vi "Write XML.vi"(9 "三级告警":string[][](array[string]), 10 "二级告警":string[][](array[string]), 11 "一级告警":string[][](array[string])) -> (0 "error out":errorcluster caption="错误输出", 3 "值":T1)   [LabVIEW 2016, in "Alarm interface.lvlib"]
uses:
  Alarm interface.lvlib
  <vilib>/Utility/xml.llb/Write to XML File(string).vi
panel:
  out "XML String":string caption="XML字符串"
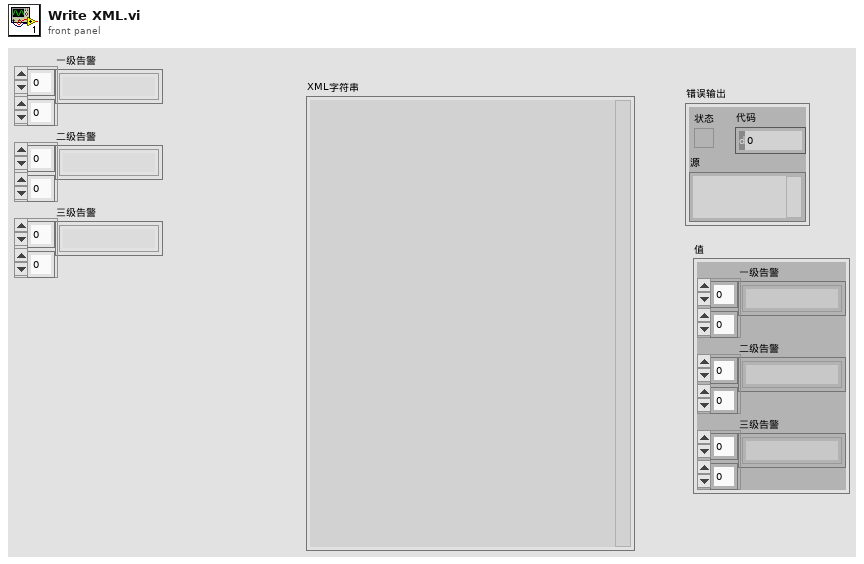
[diagram p1: front panel]
types:
  T1 = cluster{"一级告警":string[][], "二级告警":string[][], "三级告警":string[][]}
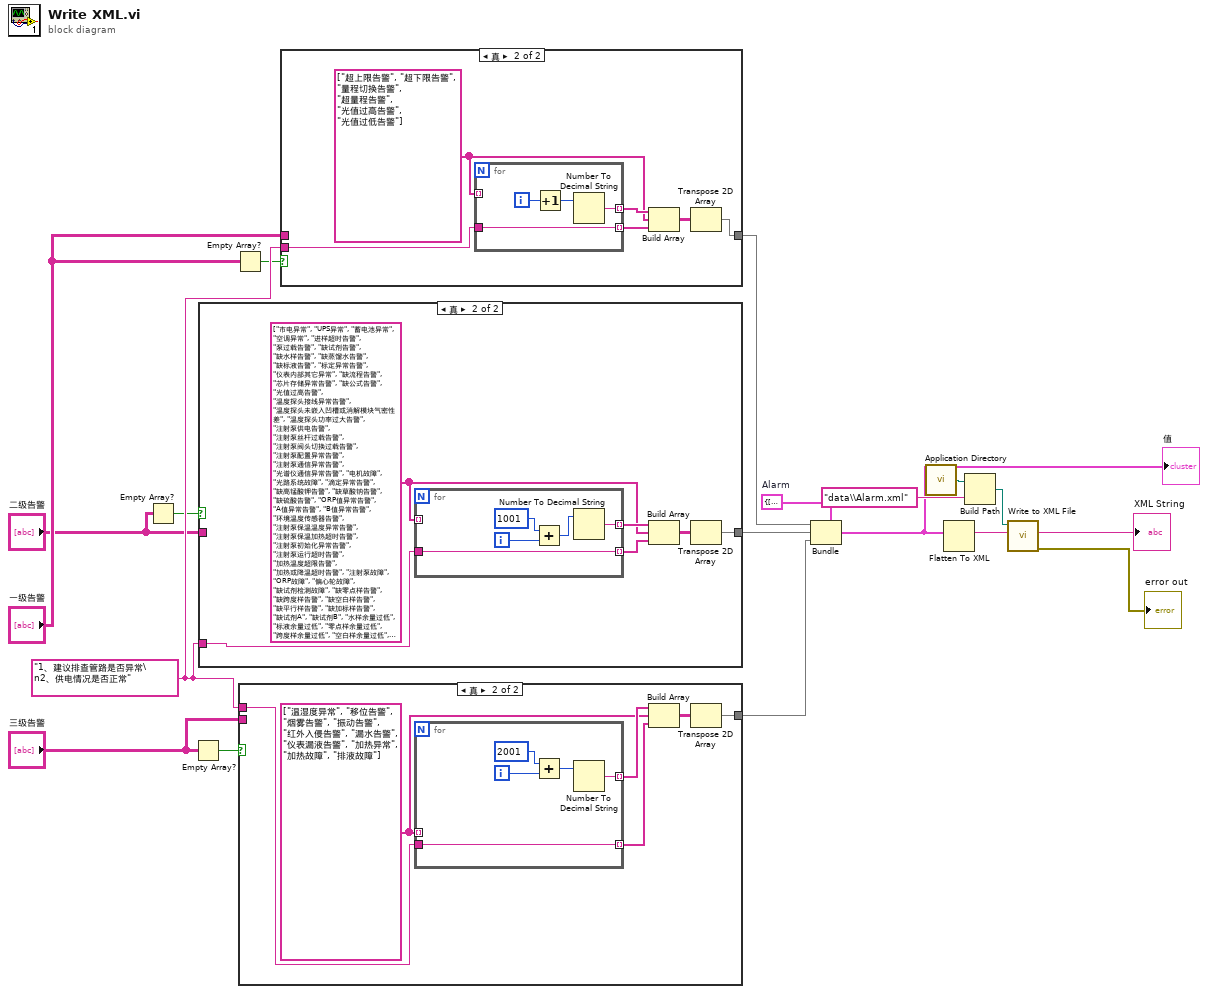
[diagram p0: block diagram]
diagram:
  w7 = "1、建议排查管路是否异常\n2、供电情况是否正常" ("分析")
  w8 = T1 {"一级告警"=[], "二级告警"=[], "三级告警"=[]}  # Alarm
  n1 = Empty Array?(array="二级告警") -> (empty?=w2:bool)
  n2 = Empty Array?(array="三级告警") -> (empty?=w4:bool)
  n3 = case shown="真" w2 {
    tunnel: [w19 w22] -> w11
    tunnel: w7 -> [_ w20]
    tunnel: "二级告警" -> [w19 _]
    frame False {
    }
    frame True {
      w23 = string[] ["市电异常", "UPS异常", "蓄电池异常", "空调异常", "进样超时告警", "泵过载告警", "缺试剂告警", "缺水样告警", "缺蒸馏水告警", "缺标液告警", "标定异常告警", "仪表内部其它异常", "缺流程告警", "芯片存储异常告警", "缺公式告警", "光值过高告警", "温度探头接线异常告警", "温度探头未嵌入凹槽或消解模块气密性差", "温度探头功率过大告警", "注射泵供电告警", "注射泵丝杆过载告警", "注射泵阀头切换过载告警", "注射泵配置异常告警", "注射泵通信异常告警", "光谱仪通信异常告警", "电机故障", "光路系统故障", "滴定异常告警", "缺高锰酸钾告警", "缺草酸钠告警", "缺硫酸告警", "ORP值异常告警", "A值异常告警", "B值异常告警", "环境温度传感器告警", "注射泵保温温度异常告警", "注射泵保温加热超时告警", "注射泵初始化异常告警", "注射泵运行超时告警", "加热温度超限告警", "加热或降温超时告警", "注射泵故障", "ORP故障", "偏心轮故障", "缺试剂检测故障", "缺零点样告警", "缺跨度样告警", "缺空白样告警", "缺平行样告警", "缺加标样告警", "缺试剂A", "缺试剂B", "水样余量过低", "标液余量过低", "零点样余量过低", "跨度样余量过低", "空白样余量过低", "平行样余量过低", "加标样余量过低", "试剂A余量过低", "试剂B余量过低", "请注意查看溶液或试剂余量并及时维护", "旋转阀通信异常告警", "旋转阀故障", "光路系统故障", "液位异常告警", "柱塞泵故障告警", "流程中断告警"] ("转置的数组")
      n4 = for {
        tunnel: w23 -> [_] mode=indexing
        tunnel: [w28] -> w24 mode=indexing
        tunnel: w20 -> [w26]
        tunnel: [w26] -> w21 mode=indexing
        i -> [w30]
        n5 = Add(x=1001, y=w30) -> (x+y=w29:i32)
        n6 = Number To Decimal String(number=w29) -> (decimal integer string=w28:string)  [unwired: 1 in]
      }
      n7 = Build Array(w24, w23, w21) -> (w25:string[][])
      n8 = Transpose 2D Array(2D array=w25) -> (transposed array=w22:string[][])
    }
  }
  n9 = Empty Array?(array="一级告警") -> (empty?=w6:bool)
  n10 = case shown="真" w4 {
    tunnel: [w31 w34] -> w9
    tunnel: w7 -> [_ w32]
    tunnel: "三级告警" -> [w31 _]
    frame False {
    }
    frame True {
      w35 = string[] ["温湿度异常", "移位告警", "烟雾告警", "振动告警", "红外入侵告警", "漏水告警", "仪表漏液告警", "加热异常", "加热故障", "排液故障"] ("转置的数组")
      n11 = for {
        tunnel: w35 -> [_] mode=indexing
        tunnel: [w40] -> w37 mode=indexing
        tunnel: w32 -> [w38]
        tunnel: [w38] -> w33 mode=indexing
        i -> [w42]
        n12 = Add(x=2001, y=w42) -> (x+y=w41:i32)
        n13 = Number To Decimal String(number=w41) -> (decimal integer string=w40:string)  [unwired: 1 in]
      }
      n14 = Build Array(w37, w35, w33) -> (w36:string[][])
      n15 = Transpose 2D Array(2D array=w36) -> (transposed array=w34:string[][])
    }
  }
  n16 = case shown="真" w6 {
    tunnel: [w43 w46] -> w12
    tunnel: w7 -> [_ w44]
    tunnel: "一级告警" -> [w43 _]
    frame False {
    }
    frame True {
      w47 = string[] ["超上限告警", "超下限告警", "量程切换告警", "超量程告警", "光值过高告警", "光值过低告警"] ("转置的数组")
      n17 = for {
        tunnel: w47 -> [_] mode=indexing
        tunnel: [w51] -> w49 mode=indexing
        tunnel: w44 -> [w50]
        tunnel: [w50] -> w45 mode=indexing
        i -> [w53]
        n18 = Increment(x=w53) -> (x+1=w52:i32)
        n19 = Number To Decimal String(number=w52) -> (decimal integer string=w51:string)  [unwired: 1 in]
      }
      n20 = Build Array(w49, w47, w45) -> (w48:string[][])
      n21 = Transpose 2D Array(2D array=w48) -> (transposed array=w46:string[][])
    }
  }
  n22 = Bundle(cluster=w8, "一级告警"=w12, "二级告警"=w11, "三级告警"=w9) -> (w10:T1)
  "值" <- w10
  n23 = call <vilib>:"Application Directory.vi"() -> ("Application Directory"=w17:path)
  n24 = Flatten To XML(anything=w10) -> (xml string=w18:string)
  n25 = Build Path(base path=w17, name or relative path="data\\Alarm.xml" ("名称或相对路径")) -> (appended path=w13:path)
  n26 = call-poly <vilib>:"Write to XML File.vi"("XML Input"=w18, "XML File Path"=w13) -> ("error out"=→"error out":errorcluster, "XML String"=→"XML String":string)  [unwired: 7 in, 1 out]
